vi "Init_UI.vi"(11 "Data ref":refnum<vi>) -> (0 "error out":errorcluster, 3 "Array Labels":string[](array[string]))   [LabVIEW 2023, in "Graph_data_collector.lvlib"]
uses:
  Graph_data_collector.lvlib
  Data Control.ctl
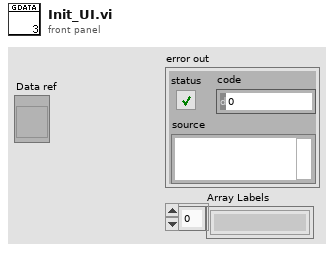
[diagram p1: front panel]
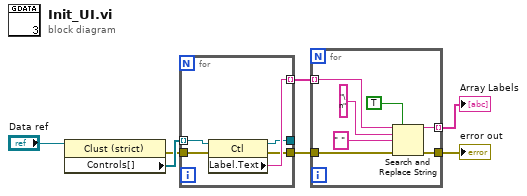
[diagram p0: block diagram]
diagram:
  n1 = property class="Clust (strict)"(reference="Data ref") -> (error out=w5:errorcluster, "Controls[]"=w6:refnum<vi>[])  [unwired: 1 in, 1 out]
  n2 = for {
    tunnel: w6 -> [w11] mode=indexing
    tunnel: [w12] -> w7 mode=indexing
    tunnel: [w10] -> w3
    tunnel: [w9] -> _
    tunnel: w5 -> [w8]
    n3 = property class="Ctl"(reference=w11, error in=w8) -> (reference out=w9:refnum<vi>, error out=w10:errorcluster, "Label.Text"=w12:string)
  }
  n4 = for {
    tunnel: w7 -> [w19] mode=indexing
    tunnel: [w17] -> w1 mode=indexing
    tunnel: w3 -> [w14]
    tunnel: [w13] -> w2
    n5 = Search and Replace String(replace all?=TRUE ("replace all? (F)"), input string=w19, search string="\n", replace string=" " ("replace string (\"\")"), error in=w14) -> (result string=w17:string, error out=w13:errorcluster)  [unwired: 3 in, 2 out]
  }
  "error out" <- w2
  "Array Labels" <- w1
